vi "format set quote prefix.vi"(8 "error in (no error)":errorcluster, 11 "format":u32) -> (0 "error out":errorcluster)   [LabVIEW 8.6]
doc: "void format_set_quote_prefix(lxw_format format);"
uses:
  pending_lvxlsxwriter/xlsxwriter.dll
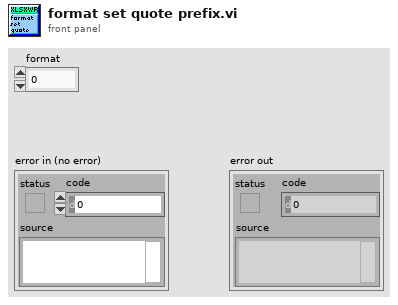
[diagram p1: front panel]
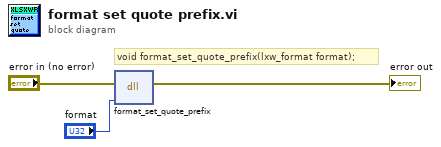
[diagram p0: block diagram]
diagram:
  # "void format_set_quote_prefix(lxw_format format);"
  n1 = dll-call lib="C:/Users/WDAGUtilityAccount/Desktop/pending_lvxlsxwriter/xlsxwriter.*" fn="format_set_quote_prefix"(error in="error in (no error)", "format"="format") -> (error out=→"error out":errorcluster)  [unwired: 4 in, 1 out]
